vi "UsrProfiles-Menu event handler.vi"(11 "ItemTag":string) -> ()   [LabVIEW 2020]
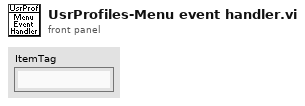
[diagram p1: front panel]
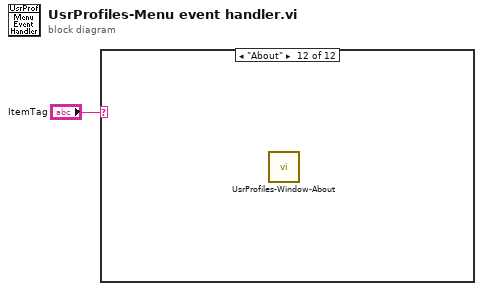
[diagram p0: block diagram]
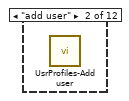
[diagram p3: hidden frame]
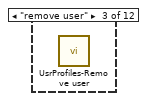
[diagram p4: hidden frame]
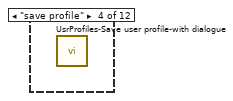
[diagram p5: hidden frame]
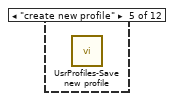
[diagram p6: hidden frame]
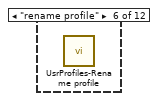
[diagram p7: hidden frame]
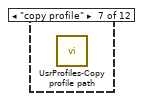
[diagram p8: hidden frame]
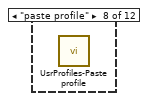
[diagram p9: hidden frame]
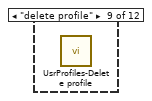
[diagram p10: hidden frame]
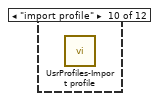
[diagram p11: hidden frame]
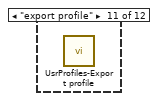
[diagram p12: hidden frame]
diagram:
  n1 = case shown="\"About\"" "ItemTag" {
    frame Default {
    }
    frame "add user" {
      n2 = call "UsrProfiles-Add user.vi"() -> ()  [unwired: 12 in]
    }
    frame "remove user" {
      n3 = call "UsrProfiles-Remove user.vi"() -> ()  [unwired: 12 in]
    }
    frame "save profile" {
      n4 = call "UsrProfiles-Save user profile-with dialogue.vi"() -> ()  [unwired: 12 in]
    }
    frame "create new profile" {
      n5 = call "UsrProfiles-Save new profile.vi"() -> ()  [unwired: 12 in]
    }
    frame "rename profile" {
      n6 = call "UsrProfiles-Rename profile.vi"() -> ()  [unwired: 12 in]
    }
    frame "copy profile" {
      n7 = call "UsrProfiles-Copy profile path.vi"() -> ()  [unwired: 12 in]
    }
    frame "paste profile" {
      n8 = call "UsrProfiles-Paste profile.vi"() -> ()  [unwired: 12 in]
    }
    frame "delete profile" {
      n9 = call "UsrProfiles-Delete profile.vi"() -> ()  [unwired: 12 in]
    }
    frame "import profile" {
      n10 = call "UsrProfiles-Import profile.vi"() -> ()  [unwired: 12 in]
    }
    frame "export profile" {
      n11 = call "UsrProfiles-Export profile.vi"() -> ()  [unwired: 12 in]
    }
    frame "About" {
      n12 = call "UsrProfiles-Window-About.vi"() -> ()  [unwired: 12 in]
    }
  }
